vi "LoadConfigFile.vi"(7 "error in (no error)":errorcluster) -> (10 "Use CGTP":bool, 12 "HTTP login":string, 14 "HTTP password":string, 15 "FTP password":string, 16 "Licensee":string, 17 "FTP user":string, 18 "Key":string, 19 "Use FTP":bool, 20 "IP":string caption="Robot IP Address", 21 "RoboguideRobotPath":path, 22 "ConnectRoboguide":bool, 23 "Use Telnet":bool, 24 "Telnet password":string, 25 "Use SNPX":bool, 27 "error out":errorcluster)   [LabVIEW 2024]
uses:
  <vilib>/Utility/config.llb/Read Key (String).vi
  <vilib>/Utility/config.llb/Read Key (Path).vi
  <vilib>/Utility/config.llb/Read Key (Boolean).vi
  <vilib>/Utility/config.llb/NI_LVConfig.lvlib
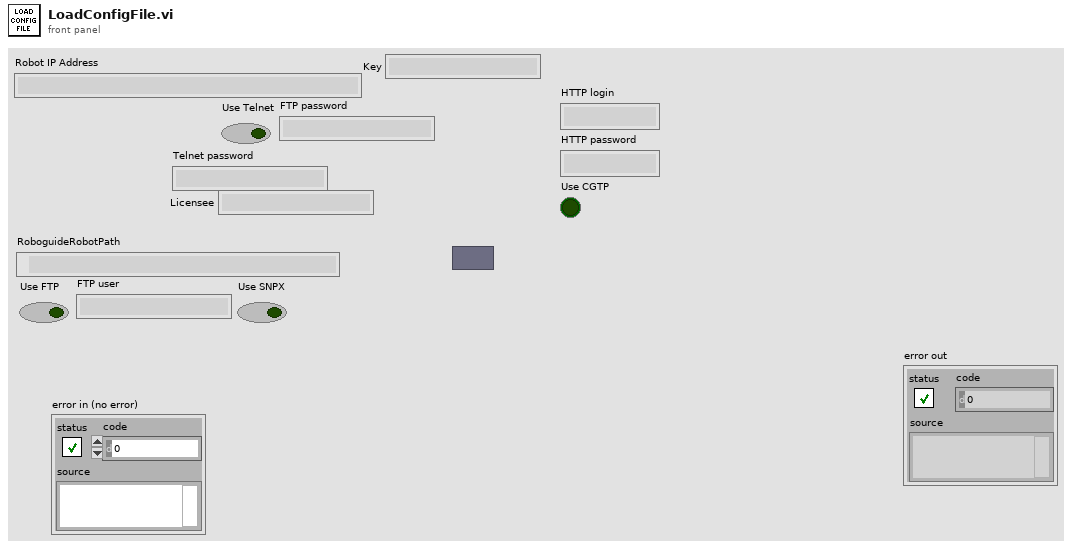
[diagram p1: front panel]
types:
  T1 = typedef "NI_LVConfig.lvlib/Config Data RefNum.ctl" = refnum<k1>
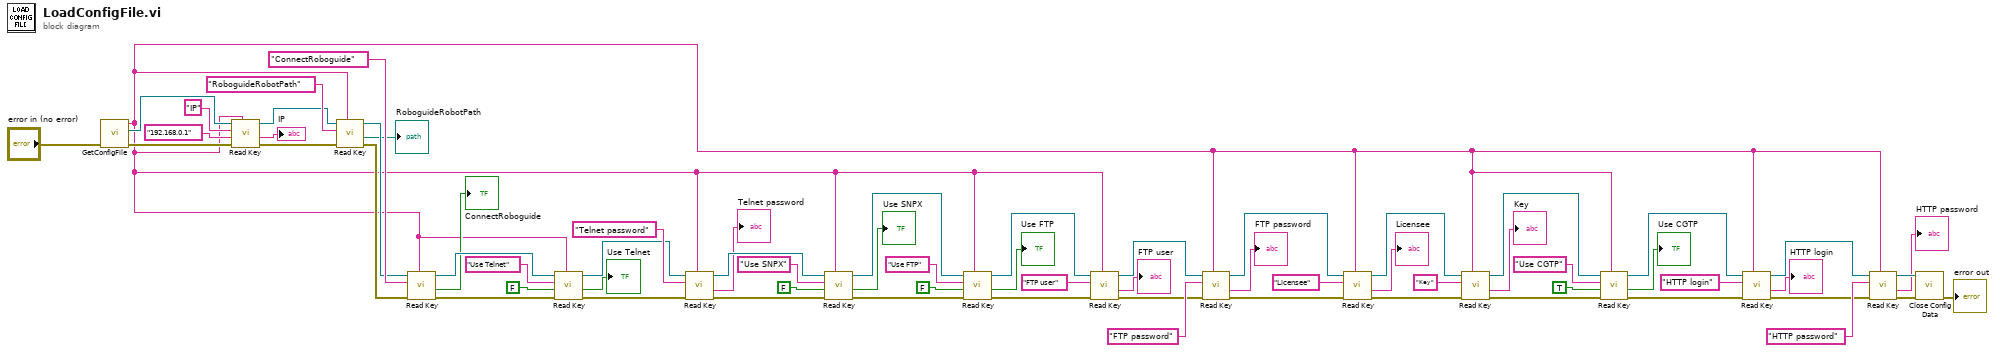
[diagram p0: block diagram]
diagram:
  n1 = call "GetConfigFile.vi"("error in (no error)"="error in (no error)") -> ("error out"=w65:errorcluster, "refnum"=w64:T1, "section"=w10:string)  [unwired: 8 in]
  n2 = call-poly <vilib>:"Read Key.vi"("section"=w10, "error in (no error)"=w65, "default value"="192.168.0.1", "key"="IP", "refnum"=w64) -> ("error out"=w45:errorcluster, "value"=→"IP":string, "refnum out"=w33:T1)  [unwired: 3 in, 1 out]
  n3 = call-poly <vilib>:"Read Key.vi"("section"=w10, "error in (no error)"=w45, "key"="RoboguideRobotPath", "refnum"=w33) -> ("error out"=w44:errorcluster, "value"=→"RoboguideRobotPath":path, "refnum out"=w34:T1)  [unwired: 4 in, 1 out]
  n4 = call-poly <vilib>:"Read Key.vi"("section"=w10, "error in (no error)"=w44, "key"="ConnectRoboguide", "refnum"=w34) -> ("error out"=w43:errorcluster, "value"=→"ConnectRoboguide":bool, "refnum out"=w46:T1)  [unwired: 4 in, 1 out]
  n5 = call-poly <vilib>:"Read Key.vi"("section"=w10, "error in (no error)"=w43, "default value"=FALSE, "key"="Use Telnet", "refnum"=w46) -> ("error out"=w42:errorcluster, "value"=→"Use Telnet":bool, "refnum out"=w47:T1)  [unwired: 3 in, 1 out]
  n6 = call-poly <vilib>:"Read Key.vi"("section"=w10, "error in (no error)"=w42, "key"="Telnet password", "refnum"=w47) -> ("error out"=w41:errorcluster, "value"=→"Telnet password":string, "refnum out"=w48:T1)  [unwired: 4 in, 1 out]
  n7 = call-poly <vilib>:"Read Key.vi"("section"=w10, "error in (no error)"=w41, "default value"=FALSE, "key"="Use SNPX", "refnum"=w48) -> ("error out"=w40:errorcluster, "value"=→"Use SNPX":bool, "refnum out"=w49:T1)  [unwired: 3 in, 1 out]
  n8 = call-poly <vilib>:"Read Key.vi"("section"=w10, "error in (no error)"=w40, "default value"=FALSE, "key"="Use FTP", "refnum"=w49) -> ("error out"=w39:errorcluster, "value"=→"Use FTP":bool, "refnum out"=w50:T1)  [unwired: 3 in, 1 out]
  n9 = call-poly <vilib>:"Read Key.vi"("section"=w10, "error in (no error)"=w39, "key"="FTP user", "refnum"=w50) -> ("error out"=w38:errorcluster, "value"=→"FTP user":string, "refnum out"=w51:T1)  [unwired: 4 in, 1 out]
  n10 = call-poly <vilib>:"Read Key.vi"("section"=w10, "error in (no error)"=w38, "key"="FTP password", "refnum"=w51) -> ("error out"=w37:errorcluster, "value"=→"FTP password":string, "refnum out"=w52:T1)  [unwired: 4 in, 1 out]
  n11 = call-poly <vilib>:"Read Key.vi"("section"=w10, "error in (no error)"=w37, "key"="Licensee", "refnum"=w52) -> ("error out"=w36:errorcluster, "value"=→"Licensee":string, "refnum out"=w53:T1)  [unwired: 4 in, 1 out]
  n12 = call-poly <vilib>:"Read Key.vi"("section"=w10, "error in (no error)"=w36, "key"="Key", "refnum"=w53) -> ("error out"=w14:errorcluster, "value"=→"Key":string, "refnum out"=w13:T1)  [unwired: 4 in, 1 out]
  n13 = call-poly <vilib>:"Read Key.vi"("section"=w10, "error in (no error)"=w14, "default value"=TRUE, "key"="Use CGTP", "refnum"=w13) -> ("error out"=w8:errorcluster, "value"=→"Use CGTP":bool, "refnum out"=w6:T1)  [unwired: 3 in, 1 out]
  n14 = call-poly <vilib>:"Read Key.vi"("section"=w10, "error in (no error)"=w8, "key"="HTTP login", "refnum"=w6) -> ("error out"=w9:errorcluster, "value"=→"HTTP login":string, "refnum out"=w5:T1)  [unwired: 4 in, 1 out]
  n15 = call-poly <vilib>:"Read Key.vi"("section"=w10, "error in (no error)"=w9, "key"="HTTP password", "refnum"=w5) -> ("error out"=w7:errorcluster, "value"=→"HTTP password":string, "refnum out"=w4:T1)  [unwired: 4 in, 1 out]
  n16 = call <vilib>:"Close Config Data.vi"("error in (no error)"=w7, "refnum"=w4) -> ("error out"=→"error out":errorcluster)  [unwired: 8 in, 1 out]
